vi "Configure for Sequential Mode.vi"(8 "error in (no error)":errorcluster, 11 "Chip Address (A2 A1 A0)":T2 max=7) -> (0 "error out":errorcluster, 3 "SPI Command":T1)   [LabVIEW 2014, in "MCP23S17.lvlib"]
doc: "Sets the chip to sequential mode (IOCON.BANK = 0)."
uses:
  MCP23S17.lvlib
  Chip Address.ctl
  SPI Command.ctl
  IOCON BANK 0 Reg Addresses.ctl
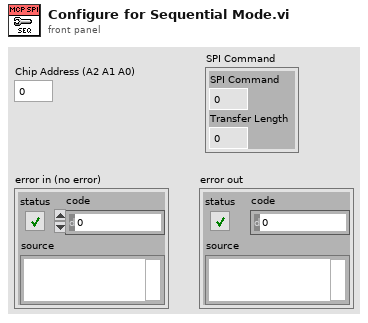
[diagram p1: front panel]
types:
  T1 = typedef "MCP23S17.lvlib/SPI Command.ctl" = cluster{"SPI Command":u32, "Transfer Length":u8}
  T2 = typedef "MCP23S17.lvlib/Chip Address.ctl" = u8
  T3 = typedef "MCP23S17.lvlib/IOCON BANK 0 Reg Addresses.ctl" = enum8{"IODIRA", "IODIRB", "IPOLA", "IPOLB", "GPINTENA", "GPINTENB", "DEFVALA", "DEFVALB", "INTCONA", "INTCONB", "IOCONA", "IOCONB", "GPPUA", "GPPUB", "INTFA", "INTFB", "INTCAPA", "INTCAPB", "GPIOA", "GPIOB", "OLATA", "OLATB"}
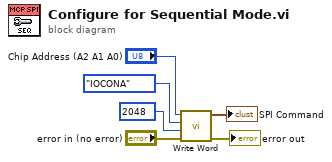
[diagram p0: block diagram]
diagram:
  n1 = call "Write Word.vi"("error in (no error)"="error in (no error)", "Value"=u16 2048, "Reg Address"=IOCON_BANK_0_Reg_Addresses."IOCONA", "Chip Address (A2 A1 A0)"="Chip Address (A2 A1 A0)") -> ("error out"=→"error out":errorcluster, "SPI Command"=→"SPI Command":T1)  [unwired: 6 in]
